vi "ReadCSV.vi"(2 "Reinit":bool, 3 "File Path (.csv)":path) -> (0 "File Open Eror":errorcluster, 1 "Data (index by row)":dbl[][](array[numeric]))   [LabVIEW 2019]
doc: "Reads data from a .csv file. Assumes a header row. Assumes indexing by row."
uses:
  <vilib>/Utility/file.llb/Read Delimited Spreadsheet (DBL).vi
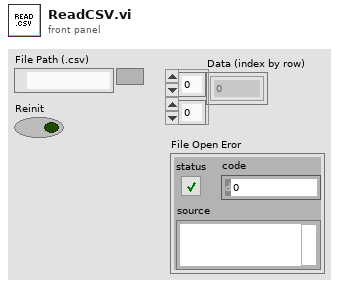
[diagram p1: front panel]
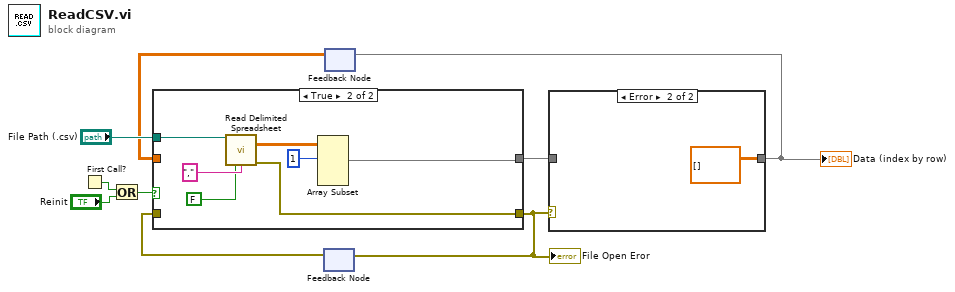
[diagram p0: block diagram]
diagram:
  n1 = First Call?() -> (First Call?: T/F=w6:bool)
  n2 = Or(x=w6, y="Reinit") -> (x .or. y?=w7:bool)
  n3 = feedback #1() -> (w1:errorcluster)  [unwired: 1 in]
  n4 = feedback #2() -> (w8:dbl[][])  [unwired: 1 in]
  n5 = case shown="True" w7 {
    tunnel: "File Path (.csv)" -> [_ w18]
    tunnel: [w11 w14] -> w4
    tunnel: w8 -> [w11 _]
    tunnel: [w10 w12] -> w2
    tunnel: w1 -> [w10 _]
    frame False {
    }
    frame True {
      n6 = call-poly <vilib>:"Read Delimited Spreadsheet.vi"("file path (dialog if empty)"=w18, "transpose? (F)"=FALSE, "delimiter (\\t)"="," ("delimiter (\\t)")) -> ("all rows"=w15:dbl[][], "error out"=w12:errorcluster)  [unwired: 7 in, 4 out]
      n7 = Array Subset(array=w15, index (row)=1 ("index")) -> (w14:dbl[][])  [unwired: 3 in]
    }
  }
  "File Open Eror" <- w2
  n8 = feedback-in #1(w2) -> ()
  n9 = case shown="Error" w2 {
    tunnel: w4 -> [w19 _]
    tunnel: [w19 dbl[][] [] ("Data (index by row)")] -> w3
    frame No Error {
    }
    frame Error {
    }
  }
  "Data (index by row)" <- w3
  n10 = feedback-in #2(w3) -> ()
